vi "BoxToRect.vi"(11 "Bounding Box":cluster{"X":dbl, "Y":dbl}[](array[cluster])) -> (2 "Array":dbl[](array[numeric]), 3 "Rectangle":T1 {"Rotation" format="%.2f"; "Left" scale=0.0..1024.0; "Right" scale=0.0..1024.0})   [LabVIEW 2019]
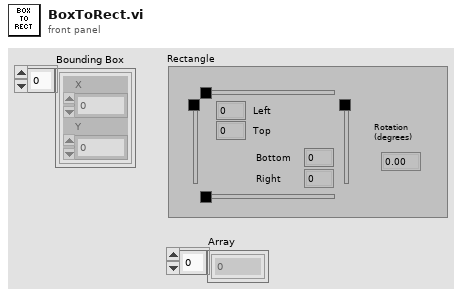
[diagram p1: front panel]
types:
  T1 = typedef "IMAQ Rectangle" = cluster{"Left":i32, "Top":i32, "Right":i32, "Bottom":i32, "Rotation":dbl}
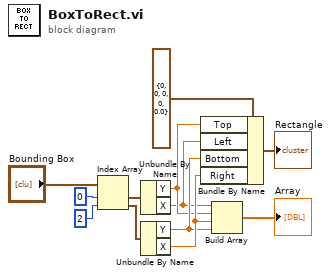
[diagram p0: block diagram]
diagram:
  n1 = Index Array(array="Bounding Box", index #1=0 ("index"), index #2=2 ("index")) -> (element #1=w4:cluster{"X":dbl, "Y":dbl}, element #2=w5:cluster{"X":dbl, "Y":dbl})
  n2 = Unbundle By Name(w4) -> ("Y"=w7:dbl, "X"=w6:dbl)
  n3 = Unbundle By Name(w5) -> ("Y"=w8:dbl, "X"=w9:dbl)
  n4 = Bundle By Name(cluster=T1 {"Left"=0, "Top"=0, "Right"=0, "Bottom"=0, "Rotation"=0.0} ("Rectangle"), "Top"=w7, "Left"=w6, "Bottom"=w8, "Right"=w9) -> (→"Rectangle":T1)
  n5 = Build Array(w6, w7, w9, w8) -> (→"Array":dbl[])
